vi "TIC Query Command daq.vi"(8 "error in (no error)":errorcluster, 10 "Command String":string, 11 "VISA Resource Name":refnum<visa-resource-name>) -> (0 "error out":errorcluster {"code" format="%.0x"}, 2 "Truncated Respose":string, 3 "VISA session (Dup)":refnum<visa-resource-name>)   [LabVIEW 2018]
doc: "Sends a command or query to the TIC, and then reads back and parses the response."
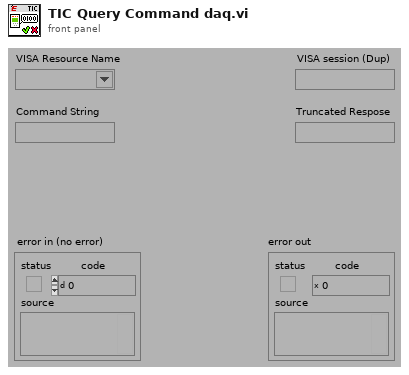
[diagram p1: front panel]
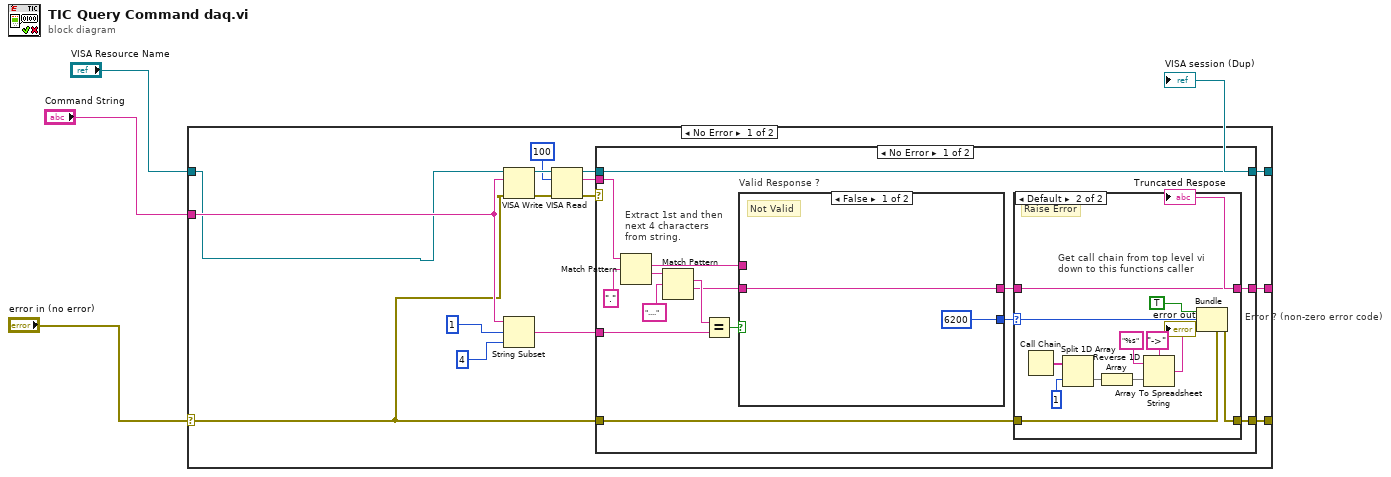
[diagram p0: block diagram]
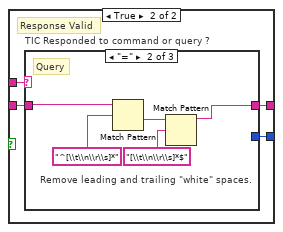
[diagram p3: hidden frame]
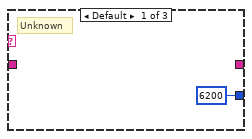
[diagram p4: hidden frame]
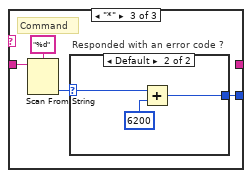
[diagram p5: hidden frame]
diagram:
  n1 = case shown="No Error" "error in (no error)" {
    selector: "error in (no error)" -> [w7 w72]
    tunnel: "VISA Resource Name" -> [w8 w73]
    tunnel: [w17 w72] -> w5
    tunnel: [w15 w73] -> w4
    tunnel: "Command String" -> [w13 _]
    tunnel: [w9 _] -> w1
    frame No Error {
      n2 = VISA Write(VISA resource name=w8, write buffer=w13, error in (no error)=w7) -> (VISA resource name out=w21:refnum<visa-resource-name>, error out=w20:errorcluster)  [unwired: 1 out]
      n3 = String Subset(string=w13, offset (0)=1, length (rest)=4 ("length (rest)")) -> (substring=w10:string)
      n4 = VISA Read(VISA resource name=w21, byte count=u32 100 ("byte count (0)"), error in (no error)=w20) -> (VISA resource name out=w16:refnum<visa-resource-name>, read buffer=w18:string, error out=w14:errorcluster)  [unwired: 1 out]
      n5 = case shown="No Error" w14 {
        selector: w14 -> [_ w70]
        tunnel: w18 -> [w34 _]
        tunnel: w7 -> [w24 _]
        tunnel: [w23 w70] -> w17
        tunnel: w16 -> [w36 w71]
        tunnel: [w36 w71] -> w15
        tunnel: w10 -> [w31 _]
        tunnel: [w22 _] -> w9
        frame No Error {
          # "Extract 1st and then\nnext 4 characters\nfrom string."
          n6 = Match Pattern(string=w34, regular expression=".") -> (match substring=w29:string, after substring=w33:string)  [unwired: 1 in, 2 out]
          n7 = Match Pattern(string=w33, regular expression="....") -> (match substring=w30:string, after substring=w28:string)  [unwired: 1 in, 2 out]
          n8 = Equal?(x=w30, y=w31) -> (x = y?=w27:bool)
          n9 = case "Valid Response ?" shown="False" w27 {
            tunnel: w29 -> [_ w56]
            tunnel: w28 -> [w52 w55]
            tunnel: [w52 w54] -> w25
            tunnel: [6200 ("code") w53] -> w26
            frame False {
              # "Not Valid"
            }
            frame True {
              # "Response Valid"
              n10 = case "TIC Responded to command or query ?" shown="\"=\"" w56 {
                tunnel: w55 -> [_ w59 w65]
                tunnel: [_ w58 _] -> w54
                tunnel: [6200 _ w63] -> w53
                frame Default {
                  # "Unknown"
                }
                frame "=" {
                  # "Remove leading and trailing \"white\" spaces."
                  # "Query"
                  n11 = Match Pattern(string=w59, regular expression="^[\\t\\n\\r\\s]*") -> (after substring=w62:string)  [unwired: 1 in, 3 out]
                  n12 = Match Pattern(string=w62, regular expression="[\\t\\n\\r\\s]*$") -> (before substring=w58:string)  [unwired: 1 in, 3 out]
                }
                frame "*" {
                  # "Command"
                  n13 = Scan From String(format string="%d", input string=w65) -> (output 1=w64:i32)  [unwired: 3 in, 3 out]
                  n14 = case "Responded with an error code ?" shown="Default" w64 {
                    selector: w64 -> [_ w68]
                    tunnel: [_ w67] -> w63
                    frame 0 {
                    }
                    frame Default {
                      n15 = Add(x=w68, y=6200) -> (x+y=w67:i32)
                    }
                  }
                }
              }
            }
          }
          n16 = case "Error ? (non-zero error code)" shown="Default" w26 {
            selector: w26 -> [_ w42]
            tunnel: w25 -> [w38 w39]
            tunnel: w24 -> [w37 w41]
            tunnel: [w37 w40] -> w23
            tunnel: [w38 w39] -> w22
            frame 0 {
              # "No Error"
            }
            frame Default {
              # "Get call chain from top level vi\ndown to this functions caller"
              # "Raise Error"
              n17 = Call Chain() -> (call chain=w46:string[])
              n18 = Split 1D Array(array=w46, index=1) -> (second subarray=w48:string[])  [unwired: 1 out]
              n19 = Reverse 1D Array(array=w48) -> (reversed array=w49:string[])
              n20 = Array To Spreadsheet String(delimiter (Tab)="->", array=w49, 3:"%s" ("format string")) -> (spreadsheet string=w43:string)
              n21 = Bundle(cluster=w41, "status"=TRUE, "code"=w42, "source"=w43) -> (w40:errorcluster)
            }
          }
        }
        frame Error {
        }
      }
    }
    frame Error {
    }
  }
  "error out" <- w5
  "Truncated Respose" <- w1
  "VISA session (Dup)" <- w4
